vi "Queque2.vi"() -> ()   [LabVIEW 2020]
panel:
  out "Numeric":dbl
  out "Waveform Chart":dbl(graph)
  in  "stop":bool
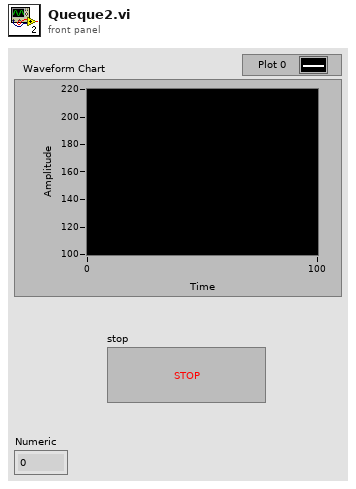
[diagram p1: front panel]
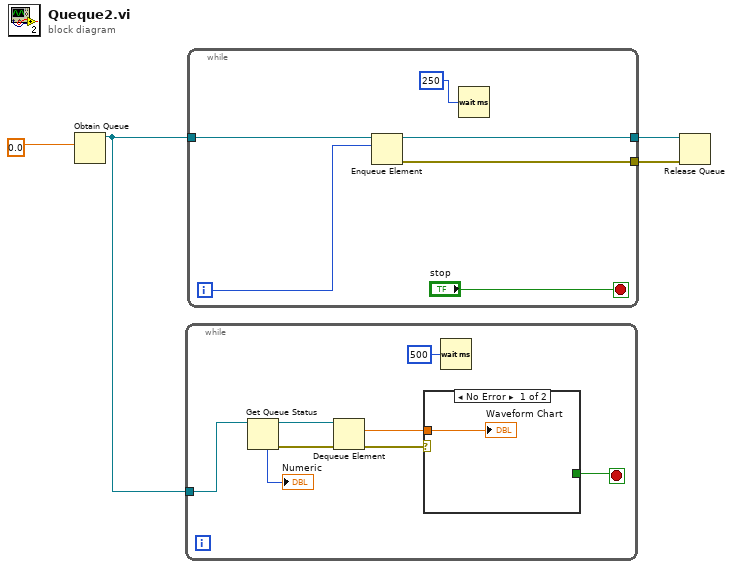
[diagram p0: block diagram]
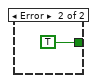
[diagram p2: hidden frame]
diagram:
  n1 = Obtain Queue(element data type=0.0) -> (queue out=w3:refnum<queue>)  [unwired: 4 in, 2 out]
  n2 = while {
    tunnel: w3 -> [w7]
    stop <- w10 stop-if-true
    n3 = Get Queue Status(queue=w7) -> (queue out=w8:refnum<queue>, error out=w5:errorcluster, # elements in queue=→"Numeric":i32)  [unwired: 2 in, 5 out]
    n4 = Dequeue Element(queue=w8, error in (no error)=w5) -> (element=w9:dbl, error out=w11:errorcluster)  [unwired: 1 in, 2 out]
    n5 = case shown="No Error" w11 {
      tunnel: [_ TRUE] -> w10
      tunnel: w9 -> [w13 _]
      frame No Error {
        "Waveform Chart" <- w13
      }
      frame Error {
      }
    }
    n6 = Wait (ms)(milliseconds to wait=u32 500) -> ()  [unwired: 1 out]
  }
  n7 = while {
    tunnel: w3 -> [w20]
    tunnel: [w19] -> w2
    tunnel: [w16] -> w1
    i -> [w18]
    stop <- "stop" stop-if-true
    n8 = Enqueue Element(queue=w20, element=w18) -> (queue out=w19:refnum<queue>, error out=w16:errorcluster)  [unwired: 2 in, 1 out]
    n9 = Wait (ms)(milliseconds to wait=u32 250) -> ()  [unwired: 1 out]
  }
  n10 = Release Queue(queue=w2, error in (no error)=w1) -> ()  [unwired: 1 in, 3 out]
